vi "Spectrogram Ridge Detection.vi"() -> ()   [LabVIEW 2023]
doc: "This example shows how to extract instantaneous frequencies of a multi-component signal by using the wavelet transform-based ridge detection algorithm. This example computes the scalogram of a signal with the WA Analytic Wavelet Transform VI and extracts the instantaneous frequency of each component by detecting the ridges in the scalogram with the WA Multiscale Ridge Detection VI. You also can use the Time Frequency Analysis VIs to compute the spectrogram of a signal and then use the WA Multiscale Ridge Detection VI to detect the ridges in the spectrogram.\n\n<b>Instructions:</b>\n1) Run this VI.\n2) Observe the <b>Ridge</b> of the <b>Scalogram</b> by using different settings."
uses:
  <vilib>/addons/Wavelet Analysis/continuous wavelet transform.llb/WA Analytic Wavelet Transform (Waveform).vi
  <vilib>/addons/_Advanced Signal Processing/NI_AdvSigProcWA.lvlib
panel:
  in  "Data":u16(ring)=104 items=["1D Example Data"=100, "-"=101, "Doppler"=102, "HOP"=103, "TF Sine"=104, "Noisy Doppler"=105, "Sea Temperature"=106, "Sp500"=107, "Power Line"=108, "Engine Knocking"=109, "HeaviSine"=110, "Bumps"=111, "Blocks"=112, "Piece Regular"=113, "HypChirps"=114, "LinChirps"=115, "Chirps"=116, "Piece Polynomial"=117, "ECG"=131, "-"=118, "2D Example Data"=119, "-"=120, "Finger Print (Image)"=121, "Iris Flower (Image)"=122, "Mammogram (Image)"=123, "Lake (Image)"=127, "Two Can 1 (Image)"=132, "Two Can 2 (Image)"=133, "Camera Man (Image)"=134]
  in  "stop":bool
  out "Ridge":u8[][](graph)
  out "Scalogram":dbl[][](graph)
  in  "Width":i32=4
  in  "Threshold ratio":dbl=0.20000000000000015 min=0.0 max=1.0 step=0.01
  # "Overview: Shows how to extract instantaneous frequencies of a multi-component signal by using the wavelet transform-based ridge detection algorithm.\nRequirements: LabVIEW Full Development System, Advanced Signal Processing Toolkit\nInstructions: \n1. Run this VI.\n2. Observe the Ridge of the Scalogram by using different settings.\n3. Click Stop to stop the VI."
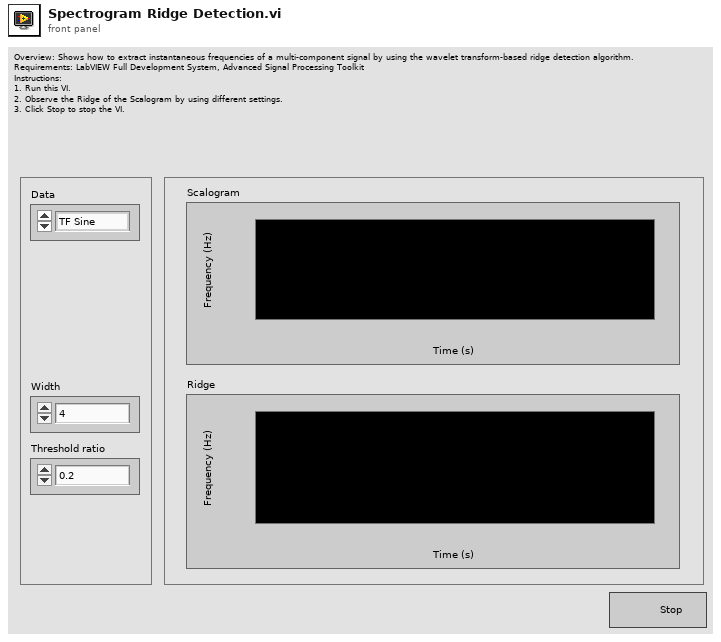
[diagram p1: front panel]
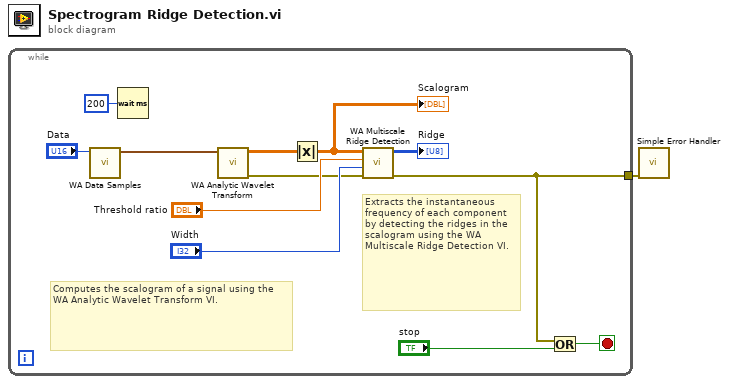
[diagram p0: block diagram]
diagram:
  n1 = while {
    tunnel: [w2] -> w1
    stop <- w7 stop-if-true
    # "Extracts the instantaneous frequency of each component by detecting the ridges in the scalogram using the WA Multiscale Ridge Detection VI."
    # "Computes the scalogram of a signal using the WA Analytic Wavelet Transform VI."
    n2 = call <vilib>:"WA Data Samples.vi"("data"="Data") -> ("signal"=w13:waveform(dbl))  [unwired: 10 out]
    n3 = Wait (ms)(milliseconds to wait=u32 200 ("millisecond multiple")) -> ()  [unwired: 1 out]
    n4 = call-poly <vilib>:"WA Analytic Wavelet Transform.vi"("signal"=w13) -> ("error out"=w3:errorcluster, "AWT coef"=w10:cdb[][])  [unwired: 3 in, 6 out]
    n5 = Absolute Value(x=w10) -> (abs(x)=w5:dbl[][])
    "Scalogram" <- w5
    n6 = call <vilib>:"WA Multiscale Ridge Detection.vi"("error in (no error)"=w3, "width"="Width", "threshold ratio"="Threshold ratio", "signal"=w5) -> ("error out"=w2:errorcluster, "ridge"=→"Ridge":u8[][])  [unwired: 6 out]
    n7 = Or(x=w2, y="stop") -> (x .or. y?=w7:bool)
  }
  n8 = call <vilib>:"Simple Error Handler.vi"("error in (no error)"=w1) -> ()  [unwired: 1 in, 8 out]
